vi "BAM Generation Create New TP Connection.vi"(2 "Allow Any SA":bool=TRUE, 5 "Data to Send":T1 {"Identifier" format="%08x"}, 7 "Source Address":u8, 11 "error in (no error)":errorcluster) -> (4 "Connection Cluster":T2 {"Packets"."Identifier" format="%08x"}, 6 "Connection Management Packet":T1 {"Identifier" format="%08x"}, 15 "error out":errorcluster)   [LabVIEW 2013, in "J1939.lvlib"]
uses:
  J1939.lvlib
  BAM Generation Connection Cluster.ctl
  API Types/CAN Outgoing Message Cluster.ctl
  Common Messages/J1939 Message TP.CM BAM.vi
  Common Messages/J1939 Message TP.DT.vi
  Frame Conversion/Convert CAN Arb ID to J1939 ID.vi
  Frame Conversion/Convert J1939 ID to CAN Arb ID.vi
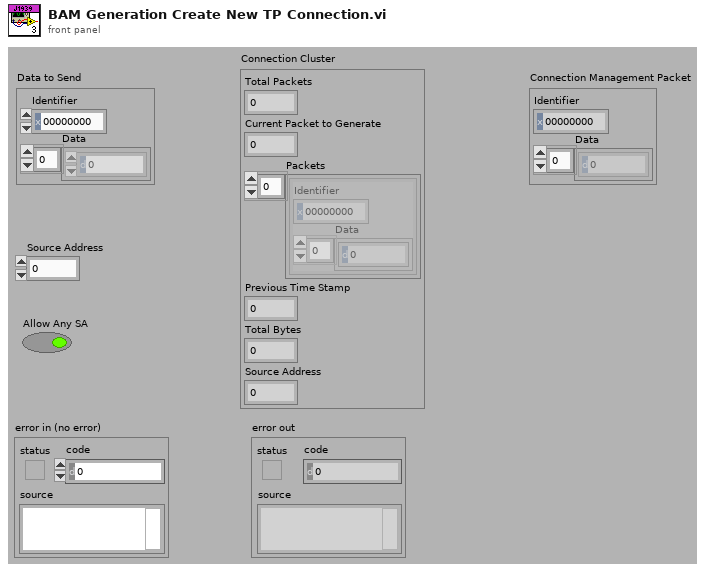
[diagram p1: front panel]
types:
  T1 = typedef "J1939.lvlib/CAN Outgoing Message Cluster.ctl" = cluster{"Identifier":u32, "Data":u8[]}
  T2 = typedef "J1939.lvlib/BAM Generation Connection Cluster.ctl" = cluster{"Total Packets":u8, "Current Packet to Generate":u8, "Packets":T1[], "Previous Time Stamp":u32, "Total Bytes":u16, "Source Address":u8}
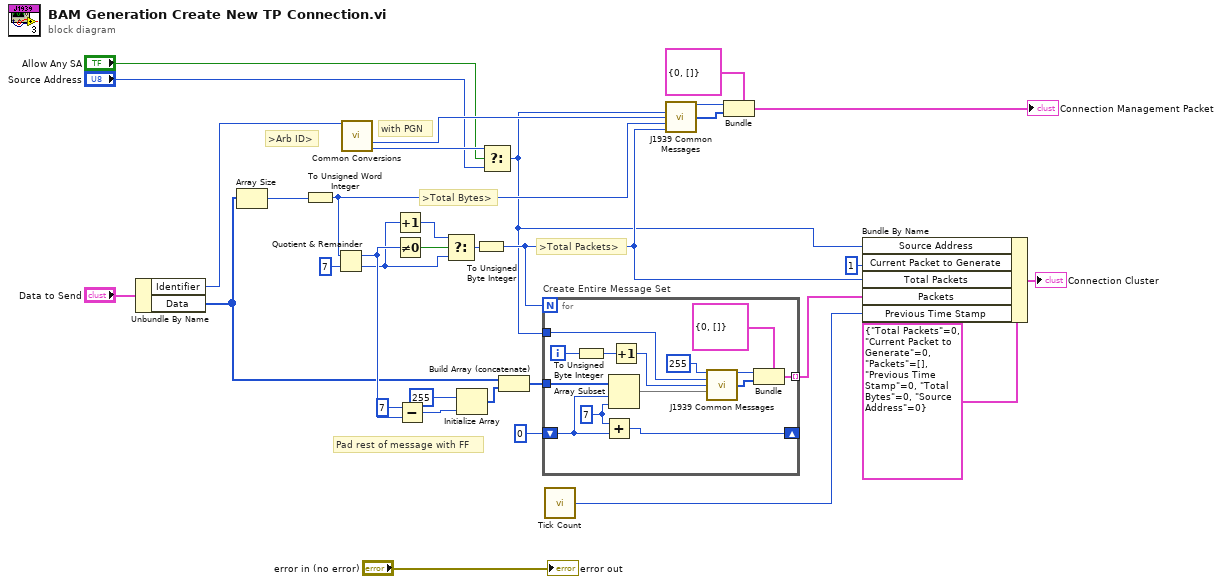
[diagram p0: block diagram]
diagram:
  # "Pad rest of message with FF"
  # ">Arb ID>"
  # "with PGN"
  # ">Total Packets>"
  # ">Total Bytes>"
  n1 = Unbundle By Name("Data to Send") -> ("Identifier"=w6:u32, "Data"=w8:u8[])
  n2 = Array Size(array=w8) -> (size(s)=w9:i32)
  n3 = To Unsigned Word Integer(number=w9) -> (unsigned 16bit integer=w15:u16)
  n4 = Quotient & Remainder(x=w15, y=u16 7) -> (x-y*floor(x/y)=w26:u16, floor(x/y)=w21:u16)
  n5 = call-poly "Common Conversions.vi"("Arb ID"=w6) -> ("PGN"=w5:u32, "Source Address"=w4:u8)  [unwired: 13 out]
  n6 = Increment(x=w21) -> (x+1=w20:u16)
  n7 = Not Equal To 0?(x=w26) -> (x != 0?=w19:bool)
  n8 = Subtract(x=u8 7, y=w26) -> (x-y=w28:u16)
  n9 = Select(t=w20, s=w19, f=w21) -> (s? t:f=w22:u16)
  n10 = Initialize Array(u8 255, w28) -> (w29:u8[])
  n11 = To Unsigned Byte Integer(number=w22) -> (unsigned 8bit integer=w31:u8)
  n12 = Select(t=w4, s="Allow Any SA", f="Source Address") -> (s? t:f=w1:u8)
  n13 = Build Array (concatenate)(w8, w29) -> (w30:u8[])
  n14 = for "Create Entire Message Set" {
    N: w31 -> [_]
    tunnel: w30 -> [w47]
    shift-right: [w44] -> _
    shift-left: 0 ("index") -> [w45]
    tunnel: [w36] -> w12 mode=indexing
    tunnel: w1 -> [w41]
    i -> [w43]
    w46 = 7 ("length")
    n15 = To Unsigned Byte Integer(number=w43) -> (unsigned 8bit integer=w42:u8)
    n16 = Add(x=w46, y=w45) -> (x+y=w44:i32)
    n17 = Array Subset(array=w47, index=w45, length=w46) -> (w35:u8[])
    n18 = Increment(x=w42) -> (x+1=w40:u8)
    n19 = call-poly "J1939 Common Messages.vi"("Destination Address"=u8 255, "Source Address"=w41, "Sequence Number"=w40, "Data"=w35) -> ("Arb ID"=w38:u32, "Data"=w37:u8[])  [unwired: 10 out]
    n20 = Bundle(cluster=T1 {"Identifier"=0, "Data"=[]}, "Identifier"=w38, "Data"=w37) -> (w36:T1)
  }
  n21 = call "Tick Count"() -> ("Tick Count(mSec)"=w13:u32)
  n22 = call-poly "J1939 Common Messages.vi"("Source Address"=w1, "PGN"=w5, "Total Message Size(bytes)"=w15, "Total Number of Packets"=w31) -> ("Arb ID"=w32:u32, "Data"=w33:u8[])  [unwired: 10 out]
  n23 = Bundle(cluster=T1 {"Identifier"=0, "Data"=[]}, "Identifier"=w32, "Data"=w33) -> (→"Connection Management Packet":T1)
  n24 = Bundle By Name(cluster=T2 {"Total Packets"=0, "Current Packet to Generate"=0, "Packets"=[], "Previous Time Stamp"=0, "Total Bytes"=0, "Source Address"=0} ("Cluster"), "Source Address"=w1, "Current Packet to Generate"=u8 1, "Total Packets"=w31, "Packets"=w12, "Previous Time Stamp"=w13) -> (→"Connection Cluster":T2)
  "error out" <- "error in (no error)"
